vi "SyncAudioTTL_SubVI.vi"(8 "External Trigger":bool, 9 "Multiplier":dbl, 10 "Filter Type":u16(ring) items=["No filter", "4k high-pass", "4k-20k band-pass", "4k-50k band-pass"], 11 "Stimulus File":path) -> (0 "error out":errorcluster, 1 "digital waveform":digitalwaveform(waveform), 2 "task out 2":refnum<k21>, 3 "Refnum out":refnum<k21>, 4 "Stim File Length (s)":dbl, 5 "Array":waveform(dbl)[](array[waveform]))   [LabVIEW 2017]
uses:
  <vilib>/DAQmx/write.llb/DAQmx Write (Analog 1D Wfm NChan NSamp).vi
  <vilib>/DAQmx/write.llb/DAQmx Write (Digital Wfm 1Chan NSamp).vi
  <vilib>/DAQmx/miscellaneous.llb/DAQmx Fill In Error Info.vi
  <vilib>/Waveform/DWDTOps.llb/DWDT Uncompress Digital.vi
  <vilib>/DAQmx/configure/timing.llb/DAQmx Timing (Sample Clock).vi
  <vilib>/DAQmx/configure/trigger.llb/DAQmx Start Trigger (Digital Edge).vi
  <vilib>/Waveform/DWDTOps.llb/DWDT Analog to Digital.vi
  <vilib>/Waveform/WDTOps.llb/WDT Number of Waveform Samples DBL.vi
  <vilib>/DAQmx/create/channels.llb/DAQmx Create Channel (AO-Voltage-Basic).vi
  <vilib>/DAQmx/create/channels.llb/DAQmx Create Channel (DO-Digital Output).vi
  <resource>/objmgr/daqmx.rc
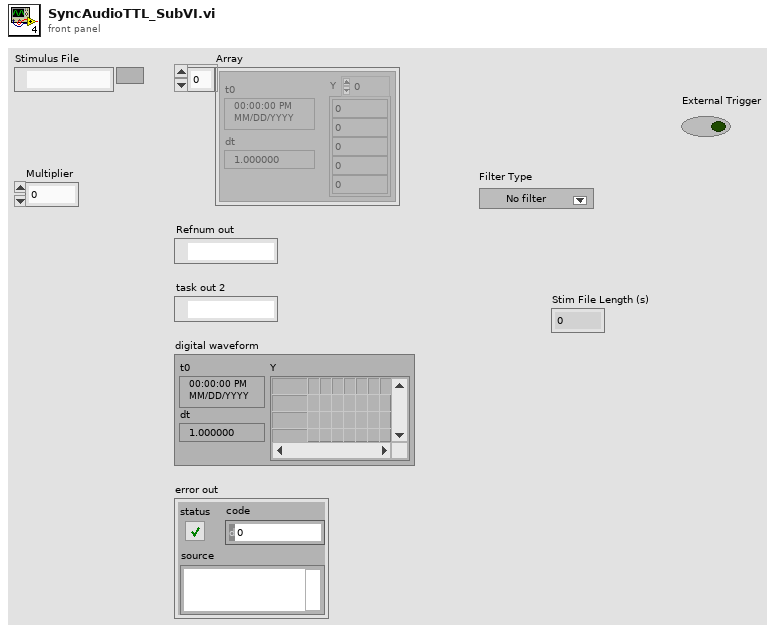
[diagram p1: front panel]
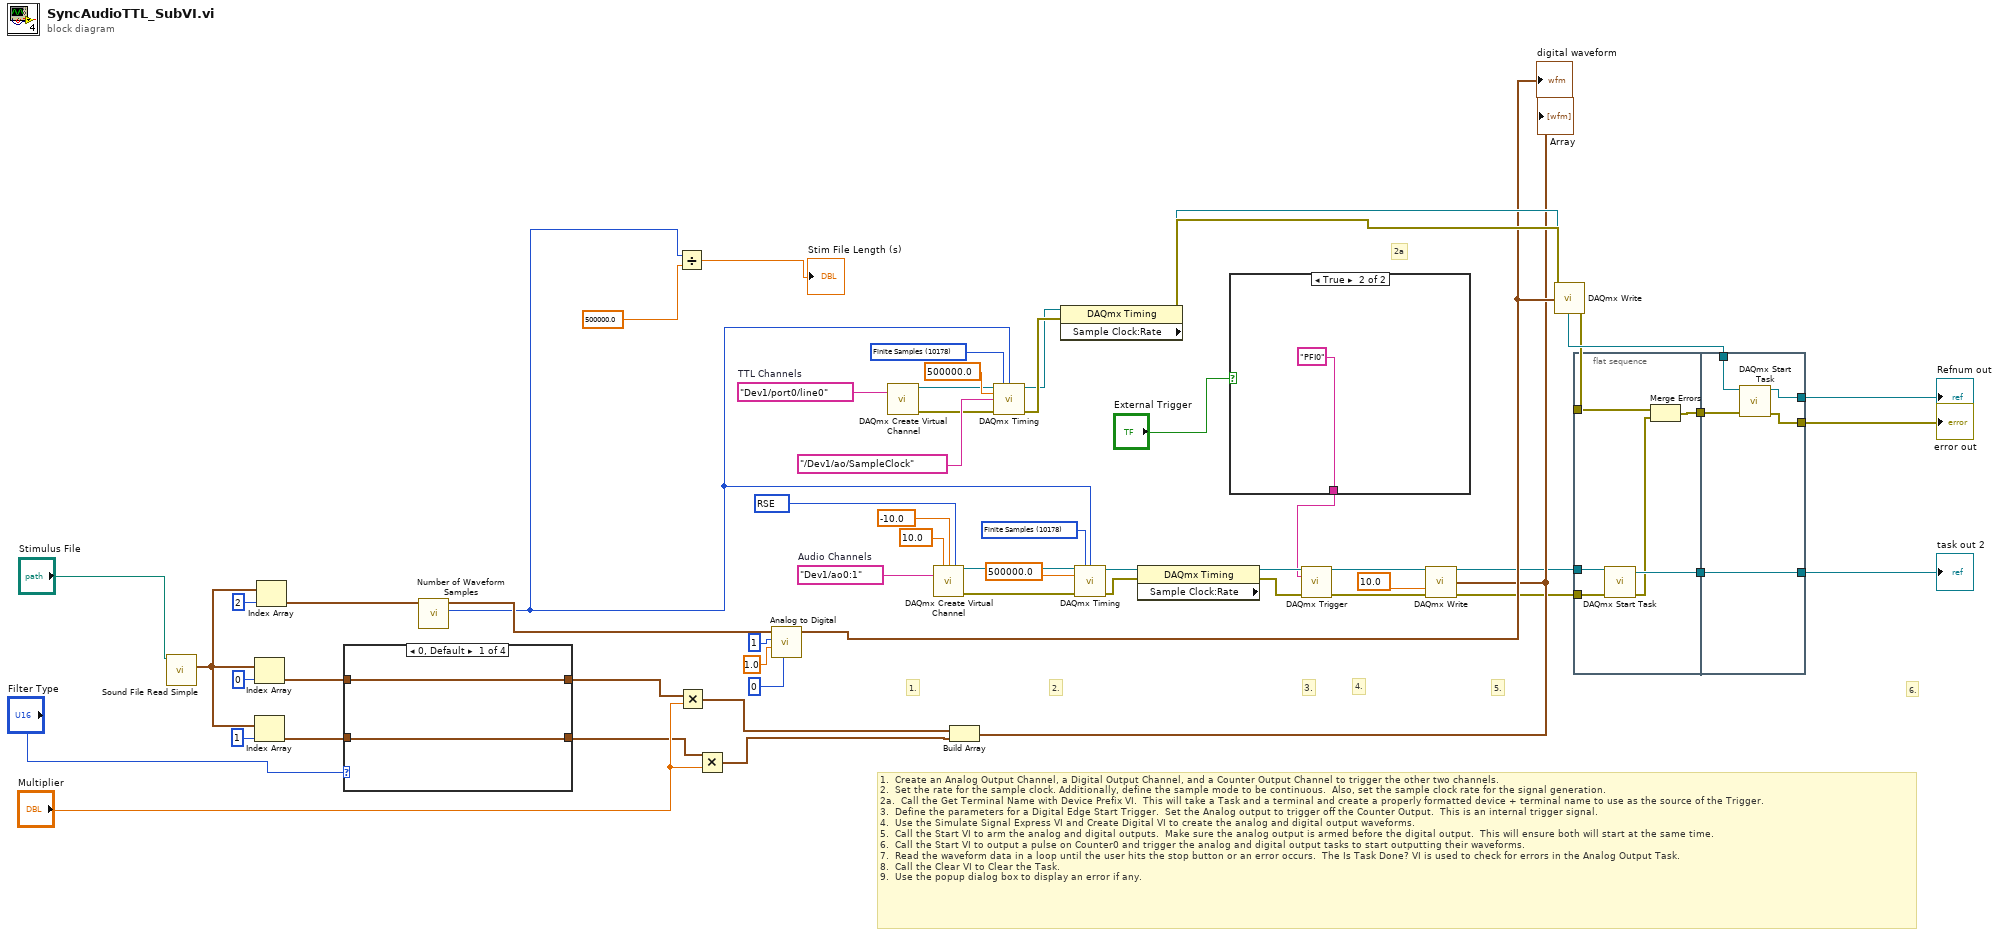
[diagram p0: block diagram]
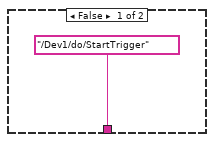
[diagram p2: hidden frame]
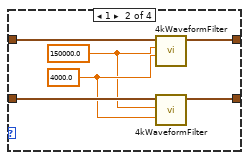
[diagram p3: hidden frame]
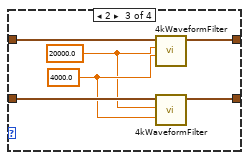
[diagram p4: hidden frame]
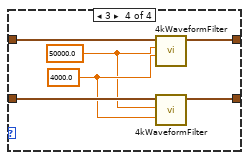
[diagram p5: hidden frame]
diagram:
  w57 = tag "Dev1/port0/line0"  # TTL Channels
  w56 = tag "Dev1/ao0:1"  # Audio Channels
  w53 = 10083 items=["Default"=-1, "RSE"=10083, "Differential"=10106, "Pseudodifferential"=12529] ("output terminal configuration")
  w12 = 10178 items=["Finite Samples"=10178, "Continuous Samples"=10123] ("sample mode")
  w7 = 10178 items=["Finite Samples"=10178, "Continuous Samples"=10123] ("sample mode")
  # "2a"
  # "6."
  # "3."
  # "4."
  # "5."
  # "1.  Create an Analog Output Channel, a Digital Output Channel, and a Counter Output Channel to trigger the other two channels.\n2.  Set the rate for the sample clock. Additionally, define the sample mode to be continuous.  Also, set the sample clock rate for the signal generation.\n2a.  Call the Get Terminal Name with Device Prefix VI.  This will take a Task and a terminal and create a properly formatted device + terminal name to use as the source of the Trigger.\n3.  Define the parameters for a Digital Edge Start Trigger.  Set the Analog output to trigger off the Counter Output.  This is an internal trigger signal.\n4.  Use the Simulate Signal Express VI and Create Digital VI to create the analog and digital output waveforms.\n5.  Call the Start VI to arm the analog and digital outputs.  Make sure the analog output is armed before the digital output.  This will ensure both will start at the same time.\n6.  Call the Start VI to output a pulse on Counter0 and trigger the analog and digital output tasks to start outputting their waveforms.\n7.  Read the waveform data in a loop until the user hits the stop button or an error occurs.  The Is Task Done? VI is used to check for errors in the Analog Output Task.\n8.  Call the Clear VI to Clear the Task.\n9.  Use the popup dialog box to display an error if any."
  # "2."
  # "1."
  n1 = call <vilib>:"Sound File Read Simple.vi"("path"="Stimulus File") -> ("data"=w34:waveform(dbl)[])  [unwired: 7 in, 3 out]
  n2 = Index Array(array=w34, index=0) -> (element=w38:waveform(dbl))
  n3 = Index Array(array=w34, index=1) -> (element=w42:waveform(dbl))
  n4 = Index Array(array=w34, index=2) -> (element=w51:waveform(dbl))
  n5 = case shown="0, Default" "Filter Type" {
    tunnel: w38 -> [w61 w67 w73 w79]
    tunnel: [w61 w66 w72 w78] -> w43
    tunnel: [w60 w65 w71 w77] -> w45
    tunnel: w42 -> [w60 w64 w70 w76]
    frame 0, Default {
    }
    frame 1 {
      w62 = 150000.0
      w63 = 4000.0
      n6 = call "4kWaveformFilter.vi"("Low cutoff"=w63, "High cutoff"=w62, "data"=w67) -> ("Waveform"=w66:waveform(dbl))  [unwired: 8 in]
      n7 = call "4kWaveformFilter.vi"("Low cutoff"=w63, "High cutoff"=w62, "data"=w64) -> ("Waveform"=w65:waveform(dbl))  [unwired: 8 in]
    }
    frame 2 {
      w68 = 20000.0
      w69 = 4000.0
      n8 = call "4kWaveformFilter.vi"("Low cutoff"=w69, "High cutoff"=w68, "data"=w73) -> ("Waveform"=w72:waveform(dbl))  [unwired: 8 in]
      n9 = call "4kWaveformFilter.vi"("Low cutoff"=w69, "High cutoff"=w68, "data"=w70) -> ("Waveform"=w71:waveform(dbl))  [unwired: 8 in]
    }
    frame 3 {
      w74 = 50000.0
      w75 = 4000.0
      n10 = call "4kWaveformFilter.vi"("Low cutoff"=w75, "High cutoff"=w74, "data"=w79) -> ("Waveform"=w78:waveform(dbl))  [unwired: 8 in]
      n11 = call "4kWaveformFilter.vi"("Low cutoff"=w75, "High cutoff"=w74, "data"=w76) -> ("Waveform"=w77:waveform(dbl))  [unwired: 8 in]
    }
  }
  n12 = call-poly <vilib>:"Number of Waveform Samples.vi"("waveform in"=w51) -> ("number of samples"=w6:i32, "waveform out"=w52:waveform(dbl))  [unwired: 8 in, 1 out]
  n13 = Divide(x=w6, y=500000.0) -> (x/y=→"Stim File Length (s)":dbl)
  n14 = Multiply(x=w43, y="Multiplier") -> (x*y=w44:waveform(dbl))
  n15 = Multiply(x=w45, y="Multiplier") -> (x*y=w46:waveform(dbl))
  n16 = call-poly <vilib>:"Analog to Digital.vi"("data format (offset binary)"=0, "full-scale range (pk-pk)"=1.0, "resolution (16 bit)"=1, "analog waveform"=w52) -> ("digital waveform"=w40:digitalwaveform)  [unwired: 4 in, 3 out]
  "digital waveform" <- w40
  n17 = call-poly <vilib>:"DAQmx Create Virtual Channel.vi"("lines"=w57) -> ("task out"=w9:refnum<k21>, "error out"=w8:errorcluster)  [unwired: 6 in, 7 out]
  n18 = call-poly <vilib>:"DAQmx Create Virtual Channel.vi"("maximum value"=10.0, "minimum value"=-10.0, "output terminal configuration"=w53, "physical channels"=w56) -> ("task out"=w13:refnum<k21>, "error out"=w14:errorcluster)  [unwired: 5 in, 5 out]
  n19 = Build Array(w44, w46) -> (w39:waveform(dbl)[])
  "Array" <- w39
  n20 = call-poly <vilib>:"DAQmx Timing.vi"("task/channels in"=w9, "sample mode"=w7, "samples per channel"=w6, "rate"=500000.0 ("Rate"), "source"=tag "/Dev1/ao/SampleClock", "error in"=w8) -> ("task out"=w27:refnum<k21>, "error out"=w30:errorcluster)  [unwired: 1 in, 7 out]
  n21 = property class="DAQmx Timing" props=["Sample Clock:Rate"](reference=w27, error in=w30) -> (reference out=w54:refnum<k21>, error out=w55:errorcluster)  [unwired: 1 out]
  n22 = call-poly <vilib>:"DAQmx Timing.vi"("task/channels in"=w13, "sample mode"=w12, "samples per channel"=w6, "rate"=500000.0, "error in"=w14) -> ("task out"=w24:refnum<k21>, "error out"=w25:errorcluster)  [unwired: 2 in, 7 out]
  n23 = property class="DAQmx Timing" props=["Sample Clock:Rate"](reference=w24, error in=w25) -> (reference out=w23:refnum<k21>, error out=w26:errorcluster)  [unwired: 1 out]
  n24 = case shown="True" "External Trigger" {
    tunnel: [tag "/Dev1/do/StartTrigger" ("source") "PFI0"] -> w1
    frame False {
    }
    frame True {
    }
  }
  n25 = call-poly <vilib>:"DAQmx Trigger.vi"("task/channels in"=w23, "source"=w1, "error in"=w26) -> ("task out"=w21:refnum<k21>, "error out"=w20:errorcluster)  [unwired: 2 in, 9 out]
  n26 = call-poly <vilib>:"DAQmx Write.vi"("task/channels in"=w21, "data"=w39, "timeout"=10.0 ("Wirite Timeout"), "error in"=w20) -> ("task out"=w18:refnum<k21>, "error out"=w19:errorcluster)  [unwired: 1 in, 9 out]
  n27 = call-poly <vilib>:"DAQmx Write.vi"("task/channels in"=w54, "data"=w40, "error in"=w55) -> ("task out"=w48:refnum<k21>, "error out"=w29:errorcluster)  [unwired: 2 in, 9 out]
  n28 = flat-sequence {
    tunnel: w18 -> [w86]
    tunnel: w19 -> [w85]
    tunnel: w29 -> [w82]
    tunnel: [w87] -> w59
    tunnel: [w83] -> w58
    tunnel: [w92] -> w15
    tunnel: w59 -> [w92]
    tunnel: w58 -> [w90]
    tunnel: w48 -> [w91]
    tunnel: [w89] -> w49
    tunnel: [w88] -> w50
    frame #0 {
      n29 = call <vilib>:"DAQmx Start Task.vi"("task/channels in"=w86, "error in"=w85) -> ("task out"=w87:refnum<k21>, "error out"=w84:errorcluster)  [unwired: 12 out]
      n30 = Merge Errors(w82, w84) -> (w83:errorcluster)
    }
    frame #1 {
      n31 = call <vilib>:"DAQmx Start Task.vi"("task/channels in"=w91, "error in"=w90) -> ("task out"=w89:refnum<k21>, "error out"=w88:errorcluster)  [unwired: 12 out]
    }
  }
  "error out" <- w50
  "Refnum out" <- w49
  "task out 2" <- w15
